vi "Delete Attribute.vi"(7 "ID":string, 8 "error in (no error)":errorcluster, 9 "Attribute":variant, 10 "Attribute Name":string, 11 "Test Executive in":refnum<class "Test Executive.lvclass">) -> (0 "error out":errorcluster, 1 "Found":bool, 3 "Test Executive out":refnum<class "Test Executive.lvclass">)   [LabVIEW 2017, in "Test Executive.lvlib" / "Test Executive.lvclass"]
uses:
  <vilib>/gpm_packages/@cs/test-executive/Source/Test Executive/TestExecutive/Test Executive.lvclass
  <vilib>/gpm_packages/@cs/test-executive/Source/Test Executive/TestExecutive/Test Executive.lvclass/Test Executive.ctl
  043b33af-864f-4ae4-bc93-78bcb832245b.vi
  <vilib>/gpm_packages/@cs/linked-list/Source/Linked List/ILinkedList/ILinked List.lvclass
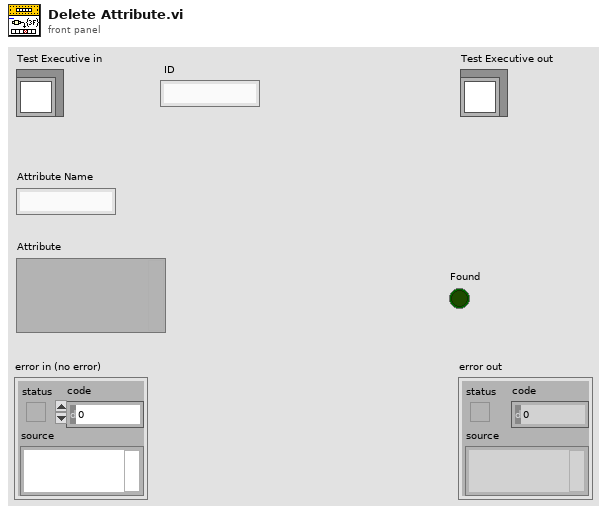
[diagram p1: front panel]
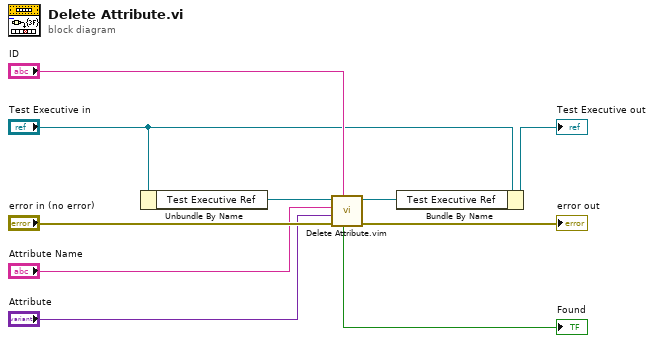
[diagram p0: block diagram]
diagram:
  n1 = Unbundle By Name("Test Executive in") -> ("Test Executive Ref"=w9:refnum<data-value>)
  n2 = call "Delete Attribute.vim"("Linked List ID"="ID", "error in (no error)"="error in (no error)", "Type"="Attribute", "Attribute Name"="Attribute Name", "Linked List Ref"=w9) -> ("error out"=→"error out":errorcluster, "Linked List Ref out"=w2:refnum<data-value>, "Found?"=→"Found":bool)  [unwired: 4 in]
  n3 = Bundle By Name(cluster="Test Executive in", "Test Executive Ref"=w2) -> (→"Test Executive out":refnum<class "Test Executive.lvclass">)
